vi "File Format Converter.vi"(8 "Error In":errorcluster, 10 "Configuration":T1={"New start time"=nan, "New end time"=nan, "Output file format"=enum."ASCII", "Save ASCII column names"=TRUE, "Prepend binary array size"=FALSE, "buffer size (-1: all)"=100000, "Channels"=[], "Group"="p", "New dt"=nan} {"buffer size (-1: all)" format="%.0p"; "New start time" format="%#_10p"}, 11 "File":path) -> (0 "Error Out":errorcluster, 2 "New file out":path, 3 "File out":path)   [LabVIEW 2016]
uses:
  Format Converter Configuration.ctl
  <vilib>/Utility/file.llb/Write Delimited Spreadsheet (DBL).vi
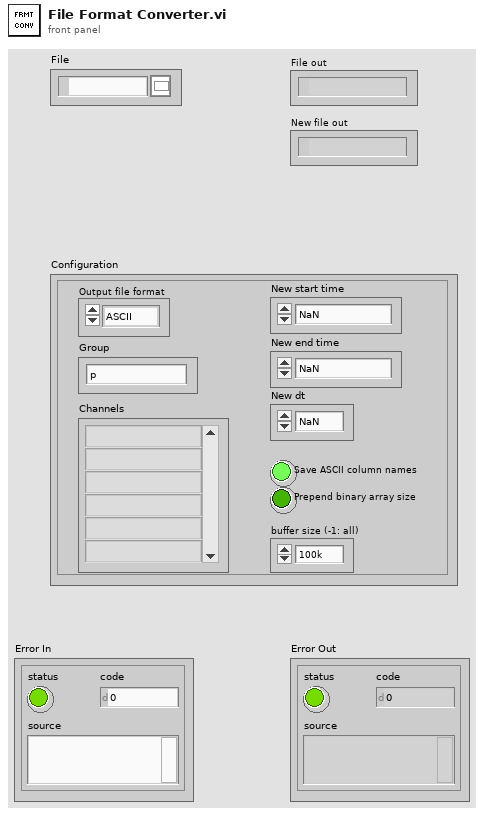
[diagram p1: front panel]
types:
  T1 = typedef "Format Converter Configuration.ctl" = cluster{"New start time":dbl, "New end time":dbl, "Output file format":enum16{"ASCII", "BINARY", "TDMS"}, "Save ASCII column names":bool, "Prepend binary array size":bool, "buffer size (-1: all)":i64, "Channels":string[], "Group":string, "New dt":dbl}
  T2 = enum16{"open", "open or create", "create or replace", "create", "open (read-only)"}
  T3 = enum16{"open", "replace", "create", "open or create", "replace or create", "replace or create with confirmation"}
  T4 = typedef "TDMS channel info.ctl" = cluster{"t0":timestamp, "dt":dbl, "Channel length":i64}
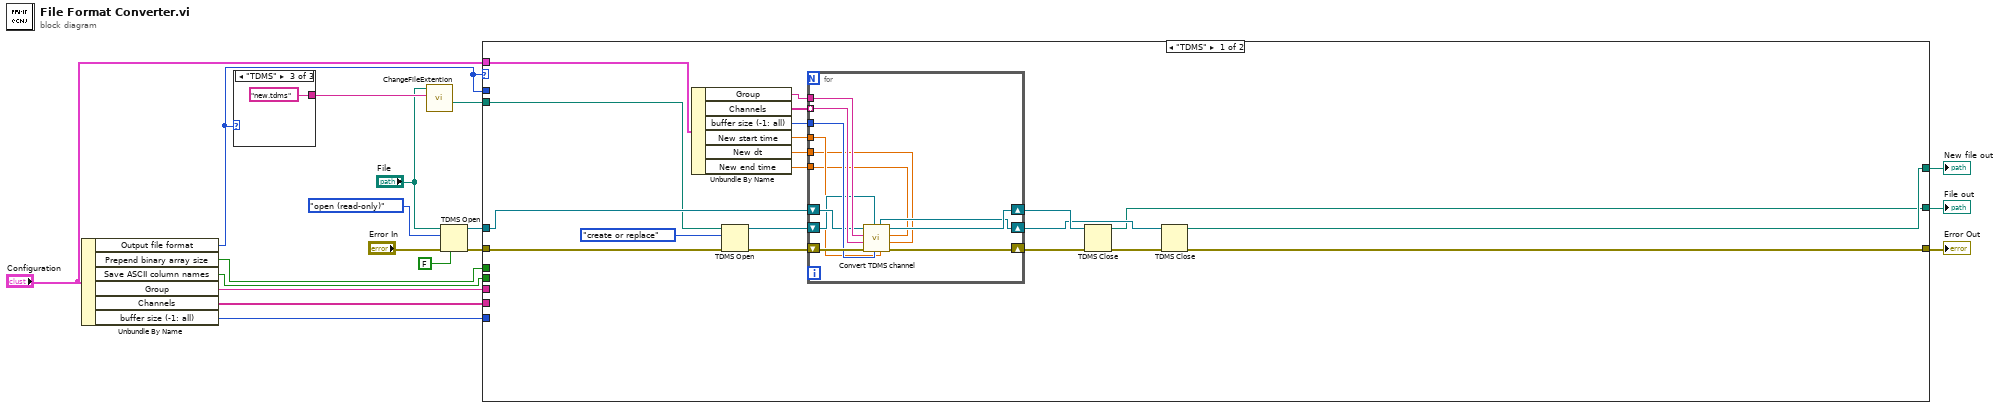
[diagram p0: block diagram]
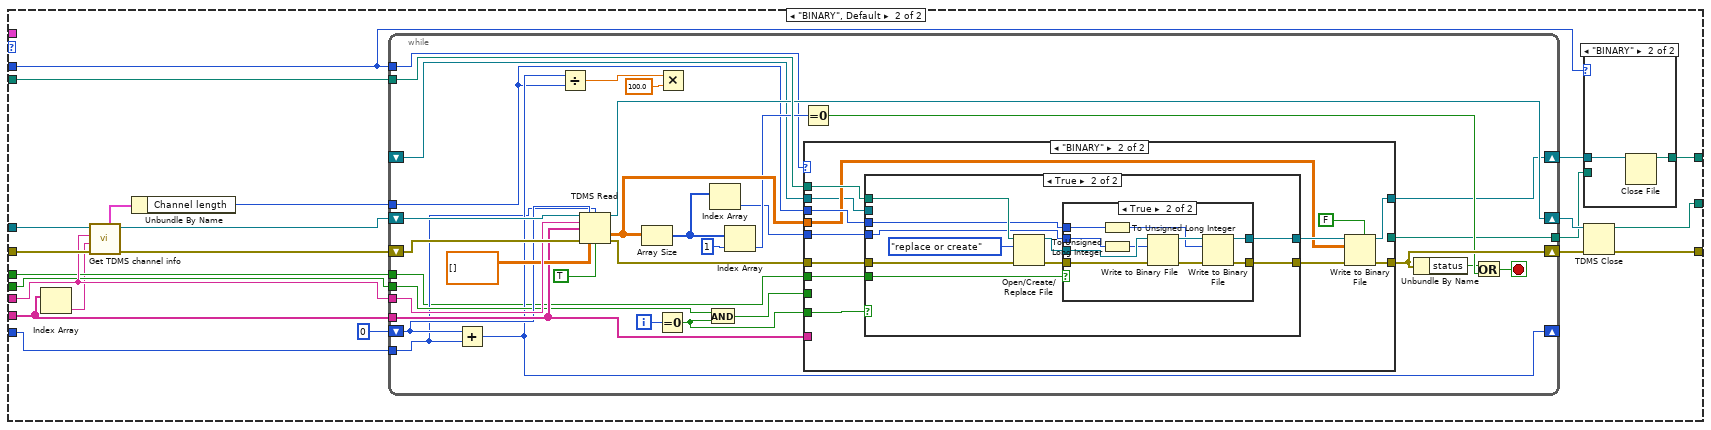
[diagram p2: hidden frame]
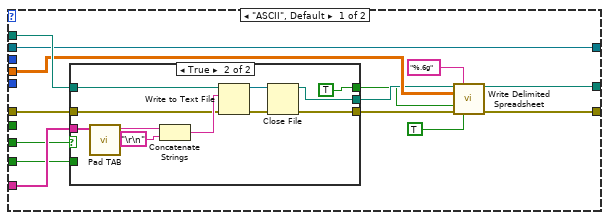
[diagram p4: hidden frame]
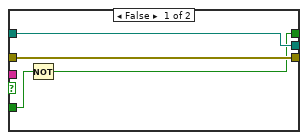
[diagram p5: hidden frame]
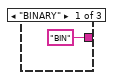
[diagram p8: hidden frame]
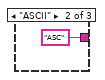
[diagram p9: hidden frame]
diagram:
  n1 = Unbundle By Name("Configuration") -> ("Output file format"=w4:enum16{"ASCII", "BINARY", "TDMS"}, "Prepend binary array size"=w6:bool, "Save ASCII column names"=w7:bool, "Group"=w9:string, "Channels"=w10:string[], "buffer size (-1: all)"=w8:i64)
  n2 = case shown="\"TDMS\"" w4 {
    tunnel: ["BIN" ("New Extention") "ASC" ("New Extention") "new.tdms" ("New Extention")] -> w14
    frame "BINARY" {
    }
    frame "ASCII" {
    }
    frame "TDMS" {
    }
  }
  n3 = call "ChangeFileExtention.vi"("New Extention"=w14, "Path"="File") -> ("Path with new extension"=w13:path)  [unwired: 5 in, 4 out]
  n4 = TDMS Open(6:FALSE ("disable buffering (T)"), 8:"Error In", 10:T2."open (read-only)" ("operation (0:open)"), 11:"File") -> (0:w18:errorcluster, 3:w17:refnum<k34>)  [unwired: 3 in]
  n5 = case shown="\"TDMS\"" w4 {
    tunnel: w18 -> [w38 w75]
    tunnel: w17 -> [w41 w74]
    tunnel: w13 -> [w39 w73]
    tunnel: [w31 w72] -> w11
    tunnel: w4 -> [_ w71]
    tunnel: w9 -> [_ w70]
    tunnel: w10 -> [_ w69]
    tunnel: w8 -> [_ w68]
    tunnel: w7 -> [_ w67]
    tunnel: w6 -> [_ w66]
    tunnel: "Configuration" -> [w27 _]
    tunnel: [w23 w56] -> w3
    tunnel: [w22 w54] -> w1
    frame "TDMS" {
      n6 = Unbundle By Name(w27) -> ("Group"=w30:string, "Channels"=w29:string[], "buffer size (-1: all)"=w28:i64, "New start time"=w26:dbl, "New dt"=w25:dbl, "New end time"=w24:dbl)
      n7 = TDMS Open(8:w38, 10:T2."create or replace" ("operation (0:open)"), 11:w39) -> (0:w36:errorcluster, 3:w37:refnum<k34>)  [unwired: 4 in]
      n8 = for {
        shift-right: [w45] -> w35
        shift-left: w36 -> [w51]
        shift-right: [w48] -> w34
        shift-left: w41 -> [w49]
        shift-right: [w46] -> w32
        shift-left: w37 -> [w47]
        tunnel: w28 -> [w50]
        tunnel: w30 -> [w53]
        tunnel: w29 -> [w52] mode=indexing
        tunnel: w26 -> [w44]
        tunnel: w25 -> [w43]
        tunnel: w24 -> [w42]
        n9 = call "Convert TDMS channel.vi"("dt"=w43, "End time"=w42, "Start time"=w44, "buffer size (-1: all)"=w50, "Output tdms ref"=w47, "Error In"=w51, "Channel name"=w52, "Group name"=w53, "Input tdms ref"=w49) -> ("Error Out"=w45:errorcluster, "Input tdms ref out"=w48:refnum<k34>, "Output tdms ref out"=w46:refnum<k34>)
      }
      n10 = TDMS Close(8:w35, 11:w34) -> (0:w33:errorcluster, 3:w22:path)
      n11 = TDMS Close(8:w33, 11:w32) -> (0:w31:errorcluster, 3:w23:path)
    }
    frame "BINARY", Default {
      n12 = Index Array(array=w69) -> (element=w61:string)  [unwired: 1 in]
      n13 = call "Get TDMS channel info.vi"("error in"=w75, "Channel name"=w61, "group name"=w70, "tdms file"=w74) -> ("error out"=w57:errorcluster, "tdms file out"=w60:refnum<k34>, "TDMS channel info"=w59:T4)  [unwired: 3 in, 2 out]
      n14 = Unbundle By Name(w59) -> ("Channel length"=w58:i64)
      n15 = while {
        tunnel: w70 -> [w110]
        tunnel: w69 -> [w107]
        tunnel: w67 -> [w100]
        tunnel: w73 -> [w106]
        shift-right: [w89] -> _
        shift-left: i64 0 -> [w103]
        shift-right: [w98] -> w63
        shift-left: w60 -> [w108]
        shift-right: [w95] -> w64
        shift-left: w57 -> [w111]
        tunnel: w58 -> [w85]
        tunnel: w71 -> [w88]
        shift-right: [w84] -> w62
        shift-left: _ -> [w83]
        tunnel: w68 -> [w81]
        tunnel: w66 -> [w80]
        tunnel: [w79] -> w55
        i -> [w102]
        stop <- w94 stop-if-true
        n16 = Add(x=w103, y=w81) -> (x+y=w89:i64)
        n17 = Divide(x=w89, y=w85) -> (x/y=w91:dbl)
        n18 = TDMS Read(0:w108, 1:w103, 2:w81, 5:w110, 7:w107, 11:w111, 12:dbl[][] [], 13:TRUE ("return channels in file order? (F)")) -> (4:w98:refnum<k34>, 10:w105:dbl[][], 15:w97:errorcluster)  [unwired: 3 out]
        n19 = Array Size(array=w105) -> (size(s)=w87:i32[])
        n20 = Equal To 0?(x=w102) -> (x = 0?=w99:bool)
        n21 = Multiply(x=w91, y=100.0) -> ()  [unwired: 1 out]
        n22 = And(x=w100, y=w99) -> (x .and. y?=w101:bool)
        n23 = Index Array(array=w87) -> (element=w86:i32)  [unwired: 1 in]
        n24 = Index Array(array=w87, index=1) -> (element=w104:i32)
        n25 = Equal To 0?(x=w104) -> (x = 0?=w93:bool)
        n26 = case shown="\"BINARY\"" w88 {
          tunnel: w107 -> [w125 _]
          tunnel: w106 -> [w124 w152]
          tunnel: w105 -> [w119 w146]
          tunnel: w101 -> [w123 _]
          tunnel: w99 -> [w122 w153]
          tunnel: w97 -> [w121 w151]
          tunnel: [w114 w145] -> w95
          tunnel: w86 -> [_ w150]
          tunnel: w85 -> [_ w149]
          tunnel: [w120 w144] -> w84
          tunnel: w83 -> [w120 w143]
          tunnel: w80 -> [_ w141]
          tunnel: [w112 _] -> w79
          frame "ASCII", Default {
            n27 = case shown="True" w123 {
              tunnel: [w126 TRUE] -> w115
              tunnel: [w128 w134] -> w113
              tunnel: w125 -> [_ w138]
              tunnel: [w129 w132] -> w116
              tunnel: w121 -> [w128 w131]
              tunnel: w124 -> [w129 w130]
              tunnel: w122 -> [w127 _]
              frame False {
                n28 = Not(x=w127) -> (.not. x?=w126:bool)
              }
              frame True {
                n29 = call "Pad TAB.vi"("Input String Array"=w138) -> ("Output String"=w139:string)  [unwired: 10 in]
                n30 = Concatenate Strings(w139, "\r\n") -> (w137:string)
                n31 = Write to Text File(file (use dialog)=w130, text=w137, error in=w131) -> (refnum out=w133:refnum<file>, error out=w135:errorcluster)  [unwired: 2 out]
                n32 = Close File(refnum=w133, error in=w135) -> (path=w132:path, error out=w134:errorcluster)
              }
            }
            n33 = call-poly <vilib>:"Write Delimited Spreadsheet.vi"("file path (dialog if empty)"=w116, "format (%.3f)"="%.6g", "2D data"=w119, "append to file? (new file:F)"=w115, "error in (no error)"=w113, "transpose? (no:F)"=TRUE) -> ("new file path (Not A Path if cancelled)"=w112:path, "error out"=w114:errorcluster)  [unwired: 8 in]
          }
          frame "BINARY" {
            n34 = case shown="True" w153 {
              tunnel: w152 -> [_ w165]
              tunnel: w151 -> [w154 w164]
              tunnel: w150 -> [_ w160]
              tunnel: w149 -> [_ w159]
              tunnel: [w154 w158] -> w148
              tunnel: [w155 w157] -> w147
              tunnel: w143 -> [w155 _]
              tunnel: w141 -> [_ w156]
              frame False {
              }
              frame True {
                n35 = Open/Create/Replace File(file path (use dialog)=w165, error in=w164, operation (0:open)=T3."replace or create") -> (refnum out=w161:refnum<file>, error out=w162:errorcluster)  [unwired: 3 in, 1 out]
                n36 = case shown="True" w156 {
                  tunnel: w162 -> [w167 w177]
                  tunnel: w161 -> [w166 w176]
                  tunnel: w160 -> [_ w175]
                  tunnel: w159 -> [_ w172]
                  tunnel: [w167 w171] -> w158
                  tunnel: [w166 w170] -> w157
                  frame False {
                  }
                  frame True {
                    n37 = To Unsigned Long Integer(number=w172) -> (unsigned 32bit integer=w168:u32)
                    n38 = To Unsigned Long Integer(number=w175) -> (unsigned 32bit integer=w169:u32)
                    n39 = Write to Binary File(file (use dialog)=w176, data=w169, error in=w177) -> (refnum out=w173:refnum<file>, error out=w174:errorcluster)  [unwired: 3 in, 1 out]
                    n40 = Write to Binary File(file (use dialog)=w173, data=w168, error in=w174) -> (refnum out=w170:refnum<file>, error out=w171:errorcluster)  [unwired: 3 in, 1 out]
                  }
                }
              }
            }
            n41 = Write to Binary File(file (use dialog)=w147, data=w146, error in=w148, 5:FALSE ("prepend array or string size? (T)")) -> (refnum out=w144:refnum<file>, error out=w145:errorcluster)  [unwired: 2 in, 1 out]
          }
        }
        n42 = Unbundle By Name(w95) -> ("status"=w92:bool)
        n43 = Or(x=w92, y=w93) -> (x .or. y?=w94:bool)
      }
      n44 = case shown="\"BINARY\"" w71 {
        tunnel: w62 -> [_ w78]
        tunnel: [w76 w77] -> w56
        tunnel: w55 -> [w76 _]
        frame "ASCII", Default {
        }
        frame "BINARY" {
          n45 = Close File(refnum=w78) -> (path=w77:path)  [unwired: 1 in, 1 out]
        }
      }
      n46 = TDMS Close(8:w64, 11:w63) -> (0:w72:errorcluster, 3:w54:path)
    }
  }
  "Error Out" <- w11
  "File out" <- w1
  "New file out" <- w3
